vi "SRV_Format Command History String.vi"(7 "Command History":string[](array[string])) -> (8 "Command History String":string)   [LabVIEW 2014]
doc: "Formats a command history string from the command history array. This is convenient for input to error messages.\n\n\nAuthor: Mike Schultz\n\n\nLogicPD, Inc\nwww.logicpd.com"
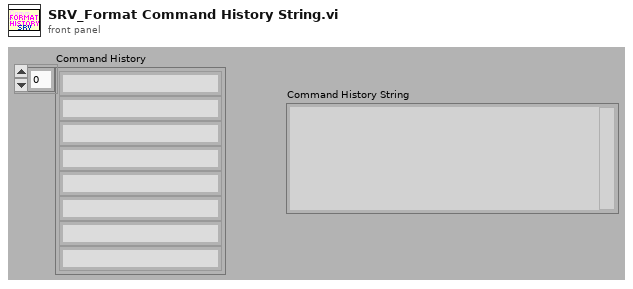
[diagram p1: front panel]
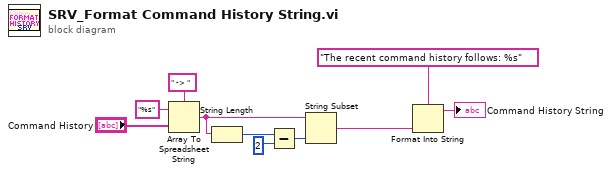
[diagram p0: block diagram]
diagram:
  n1 = Array To Spreadsheet String(delimiter (Tab)=" -> " ("Element Separator(, )"), array="Command History", 3:"%s" ("format string")) -> (spreadsheet string=w8:string)
  n2 = String Length(string=w8) -> (length=w5:i32)
  n3 = Subtract(x=w5, y=2) -> (x-y=w7:i32)
  n4 = String Subset(string=w8, length (rest)=w7) -> (substring=w1:string)  [unwired: 1 out]
  n5 = Format Into String(format string="The recent command history follows: %s", w1) -> (resulting string=→"Command History String":string)  [unwired: 2 in, 1 out]
